vi "Test  JSON subitems in Variant.vi"() -> ()   [LabVIEW 2011]
doc: "Demonstrates the use of the Variant JSON VIs for converting to and from a complex cluster."
uses:
  JSON Value/JSON Value.lvclass
  JSON Value/Set from JSON string.vi
  JSON Value/Get as JSON string.vi
  Variant JSON/Get as Variant.vi
  Variant JSON/Variant to JSON.vi
  JSON Value/Get Item by name array.vi
  Get Polymorphic/JSON GetSet.lvlib
  Variant JSON/Variant JSON.lvlib
panel:
  out "lossless":bool
  out "Filled cluster":T1
  in  "Static data structure definition":T1
  out "Variant out":variant
  out "Recreated JSON":string
  in  "Incoming JSON":string="{\"Regular String\": \"test\",\n\"Array\":[{\"type\":\"SimMultimeter\",\"config\":{\"maxV\":10,\"maxI\":5}},123,[6,7,\"eight\"]],\n\"subitem\":[\"test\",null,\"test2\",123],\n\"2nd Array\":[{\"type\":\"SimMultimeter\",\"config\":{\"maxV\":10,\"maxI\":5}},123,[6,7,\"eight\"]],\n\"2nd subitem\":[\"test\",null,\"test2\",123]\n\n}"
  # "Experiments in using JSON to hold configurations for application subcomponents, where the application code does not depend on the exact structure of the config past to the subcomponents."
  # "Two versions:\n1) strings with names \"Tagged\" with <JSON> at start.\n2) JSON class objects"
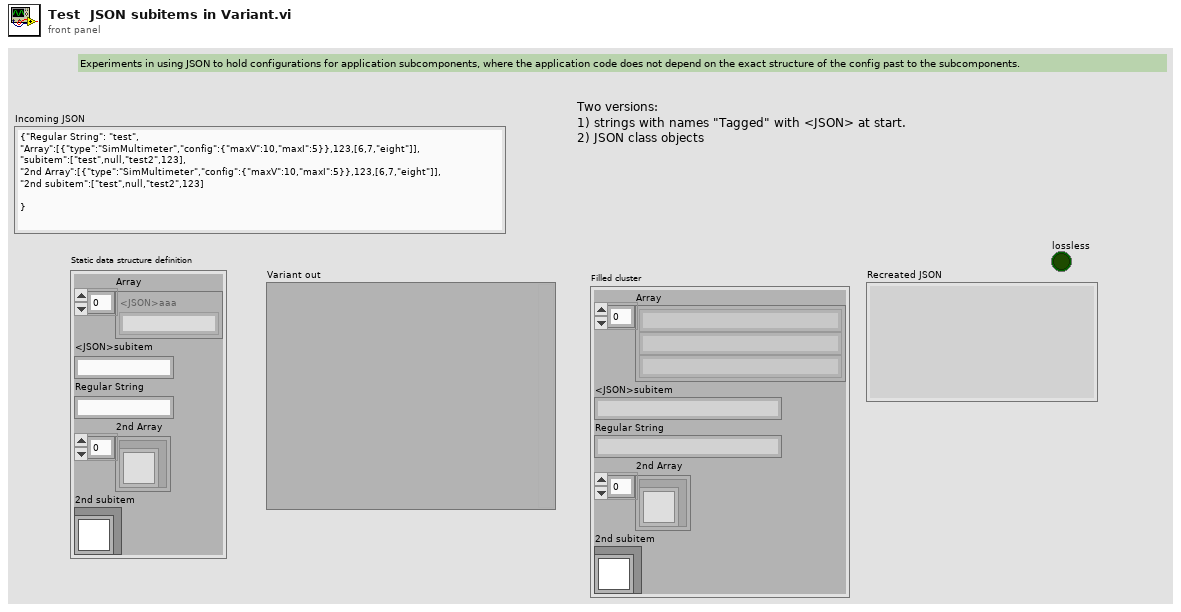
[diagram p1: front panel]
types:
  T1 = cluster{"Array":string[], "<JSON>subitem":string, "Regular String":string, "2nd Array":refnum<class "JSON Value.lvclass">[], "2nd subitem":refnum<class "JSON Value.lvclass">}
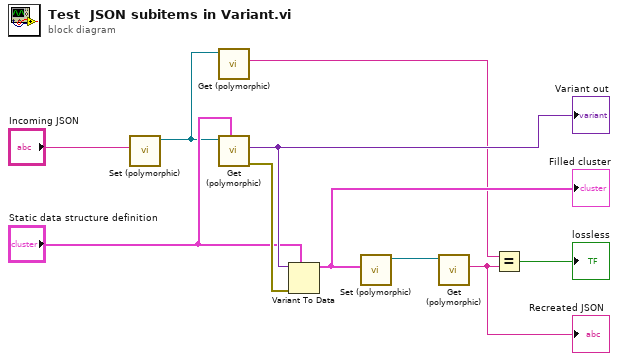
[diagram p0: block diagram]
diagram:
  n1 = call-poly "Set (polymorphic).vi"("JSON stream"="Incoming JSON") -> ("JSON Value out"=w4:refnum<class "JSON Value.lvclass">)  [unwired: 8 in, 2 out]
  n2 = call-poly "Get (polymorphic).vi"("JSON Value in"=w4) -> ("String"=w3:string)  [unwired: 9 in, 1 out]
  n3 = call-poly "Get (polymorphic).vi"("Variant (Data Type)"="Static data structure definition", "JSON in"=w4) -> ("error out"=w8:errorcluster, "Variant out"=w9:variant)  [unwired: 7 in, 1 out]
  "Variant out" <- w9
  n4 = Variant To Data(error in=w8, type="Static data structure definition", Variant=w9) -> (data=w7:T1)  [unwired: 1 out]
  "Filled cluster" <- w7
  n5 = call-poly "Set (polymorphic).vi"("Variant"=w7) -> ("JSON Value out"=w5:refnum<class "JSON Value.lvclass">)  [unwired: 9 in, 1 out]
  n6 = call-poly "Get (polymorphic).vi"("JSON Value in"=w5) -> ("String"=w2:string)  [unwired: 9 in, 1 out]
  "Recreated JSON" <- w2
  n7 = Equal?(x=w3, y=w2) -> (x = y?=→"lossless":bool)
